vi "main.vi"() -> ()   [LabVIEW 2017]
panel:
  out "All rows sortedd":dbl[][](array[numeric])
  out "replaced row array":dbl[][](array[numeric])
  out "sorted row":dbl[](array[numeric])
  in  "index (row)":i32
  out "Array":dbl[][](array[numeric])
  in  "Rows":i32
  in  "Cols":i32
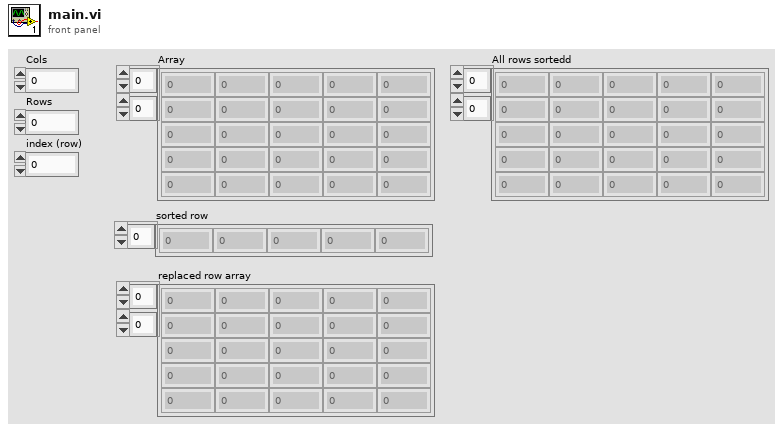
[diagram p1: front panel]
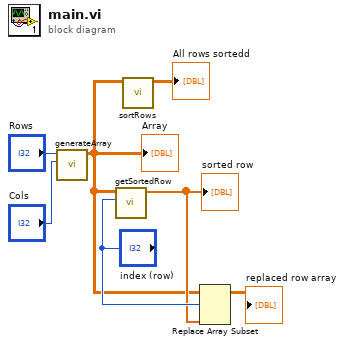
[diagram p0: block diagram]
diagram:
  n1 = call "generateArray.vi"("Cols"="Cols", "Rows"="Rows") -> ("Array"=w2:dbl[][])  [unwired: 9 in]
  "Array" <- w2
  n2 = call "getSortedRow.vi"("index (row)"="index (row)", "Array"=w2) -> ("sorted array"=w4:dbl[])  [unwired: 9 in]
  "sorted row" <- w4
  n3 = call "sortRows.vi"("Array in"=w2) -> ("Array out"=→"All rows sortedd":dbl[][])  [unwired: 10 in]
  n4 = Replace Array Subset(array=w2, new element=w4, index (row)="index (row)") -> (→"replaced row array":dbl[][])  [unwired: 1 in]
